vi "LVClass_CameraSet Get Files Destination.vi"(0 "CameraSet in":refnum<class "CameraSet.lvclass">, 5 "repertoire":path, 11 "error in (no error)":errorcluster) -> (4 "CameraSet out":refnum<class "CameraSet.lvclass">, 15 "error out":errorcluster)   [LabVIEW 2020, in "CameraSet.lvclass"]
uses:
  CameraSet.lvclass
  CameraSet.lvclass/CameraSet.ctl
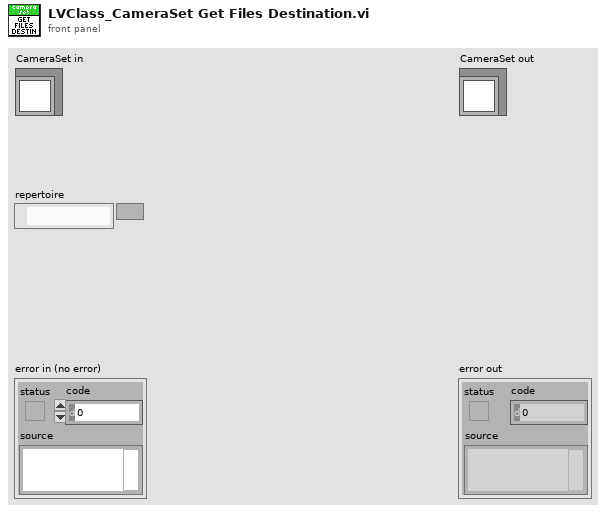
[diagram p1: front panel]
types:
  T1 = typedef "CameraSpecifications.ctl" = cluster{"Grabber name":string, "Camera name":string, "Camera sn":string, "Pixels_um":T2, "Maximum level":u32, "Data alignment":T5, "Is signed":bool, "Acquisition start":T3, "Acquisition length":T3, "MaxFrameRate_Hz":sgl, "Chip type":enum16{"Progressive scan", "Frame transfert"}}
  T2 = typedef "General dimensions definition.ctl" = cluster{"Size":T3, "Step":T4}
  T3 = typedef "Point2D.ctl" = cluster{"X":u32, "Y":u32}
  T4 = typedef "Point2Df.ctl" = cluster{"X":sgl, "Y":sgl}
  T5 = typedef "Data alignment enum.ctl" = enum16{"8", "16", "32"}
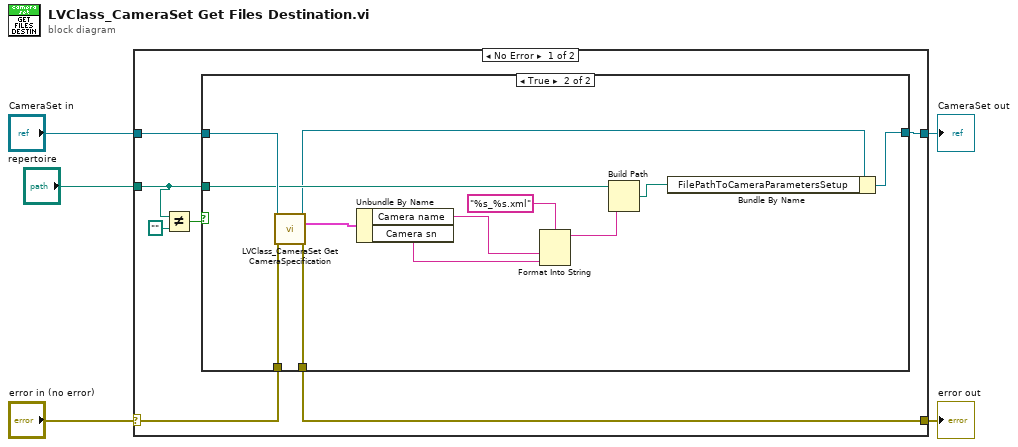
[diagram p0: block diagram]
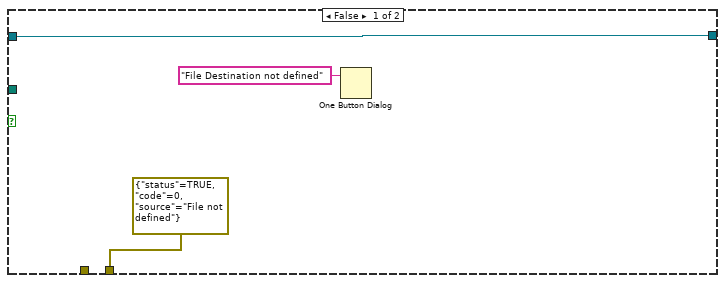
[diagram p2: hidden frame]
diagram:
  n1 = case shown="No Error" "error in (no error)" {
    selector: "error in (no error)" -> [w12 w29]
    tunnel: [w11 w29] -> w4
    tunnel: [w9 w28] -> w2
    tunnel: "CameraSet in" -> [w10 w28]
    tunnel: "repertoire" -> [w6 _]
    frame No Error {
      n2 = Not Equal?(x=w6, y=path "") -> (x != y?=w7:bool)
      n3 = case shown="True" w7 {
        tunnel: w12 -> [_ w27]
        tunnel: [errorcluster {"status"=TRUE, "code"=0, "source"="File not defined"} ("error out") w26] -> w11
        tunnel: w10 -> [w13 w25]
        tunnel: w6 -> [_ w23]
        tunnel: [w13 w21] -> w9
        frame False {
          n4 = One Button Dialog(message="File Destination not defined") -> ()  [unwired: 1 in, 1 out]
        }
        frame True {
          n5 = call "LVClass_CameraSet Get CameraSpecification.vi"("CameraSet.lvclass"=w25, "error in (no error)"=w27) -> ("CameraSet.lvclass"=w22:refnum<class "CameraSet.lvclass">, "Camera Config"=w24:T1, "error out"=w26:errorcluster)  [unwired: 11 in]
          n6 = Unbundle By Name(w24) -> ("Camera name"=w18:string, "Camera sn"=w17:string)
          n7 = Format Into String(format string="%s_%s.xml", w18, w17) -> (resulting string=w16:string)  [unwired: 2 in, 1 out]
          n8 = Build Path(base path=w23, name or relative path=w16) -> (appended path=w20:path)
          n9 = Bundle By Name(cluster=w22, "FilePathToCameraParametersSetup"=w20) -> (w21:refnum<class "CameraSet.lvclass">)
        }
      }
    }
    frame Error {
    }
  }
  "error out" <- w4
  "CameraSet out" <- w2
